vi "S2C_VAR_BuildArray.vi"(7 "Type":string(combo), 8 "Error In":errorcluster, 10 "Size":i32, 11 "Name":string) -> (0 "Error Out":errorcluster, 3 "Array":T1(array[cluster]))   [LabVIEW 2015]
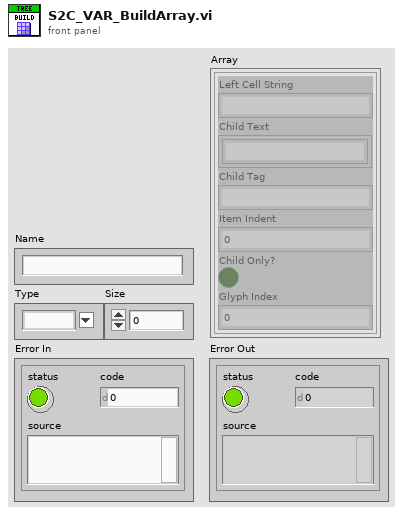
[diagram p1: front panel]
types:
  T1 = cluster{"Left Cell String":string, "Child Text":string[], "Child Tag":string, "Item Indent":i32, "Child Only?":bool, "Glyph Index":i32}[]
  T2 = cluster{"Left Cell String":string, "Child Text":string[], "Child Tag":string, "Item Indent":i32, "Child Only?":bool, "Glyph Index":i32}
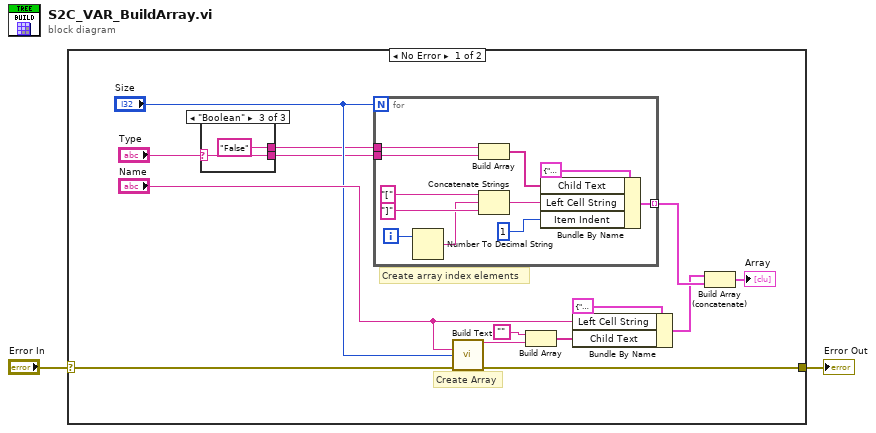
[diagram p0: block diagram]
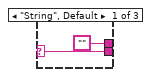
[diagram p2: hidden frame]
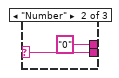
[diagram p3: hidden frame]
diagram:
  n1 = case shown="No Error" "Error In" {
    selector: "Error In" -> [w12 w34]
    tunnel: [w7 w34] -> w1
    frame No Error {
      # "Create array index elements"
      # "Create Array"
      n2 = case shown="\"Boolean\"" "Type" {
        selector: "Type" -> [w17 w20 w22]
        tunnel: [w17 w20 w22] -> w5
        tunnel: ["" "0" "False"] -> w4
        frame "String", Default {
        }
        frame "Number" {
        }
        frame "Boolean" {
        }
      }
      n3 = for {
        N: "Size" -> [_]
        tunnel: [w28] -> w9 mode=indexing
        tunnel: w5 -> [w24]
        tunnel: w4 -> [w23]
        i -> [w31]
        n4 = Number To Decimal String(number=w31) -> (decimal integer string=w30:string)  [unwired: 1 in]
        n5 = Build Array(w23, w24) -> (w27:string[])
        n6 = Concatenate Strings("[", w30, "]" ("string")) -> (w26:string)
        n7 = Bundle By Name(cluster=T2 {"Left Cell String"="", "Child Text"=[], "Child Tag"="", "Item Indent"=0, "Child Only?"=TRUE, "Glyph Index"=0} ("Item"), "Child Text"=w27, "Left Cell String"=w26, "Item Indent"=1) -> (w28:T2)
      }
      n8 = call "Build Text"("Name"="Name", "Cnt"="Size", "error in (no error)"=w12) -> ("Result"=w14:string, "error out"=w7:errorcluster)  [unwired: 11 in]
      n9 = Build Array("", w14) -> (w13:string[])
      n10 = Bundle By Name(cluster=T2 {"Left Cell String"="", "Child Text"=["", ""], "Child Tag"="", "Item Indent"=0, "Child Only?"=FALSE, "Glyph Index"=0} ("Item"), "Left Cell String"="Name", "Child Text"=w13) -> (w8:T2)
      n11 = Build Array (concatenate)(w8, w9) -> (→"Array":T1)
    }
    frame Error {
    }
  }
  "Error Out" <- w1
